vi "pf_Get DLL Path.vi"(8 "error in (no error)":errorcluster) -> (0 "error out":errorcluster, 3 "DLL path":path)   [LabVIEW 2025, in "Photonfocus_Toolkit.lvlib"]
uses:
  Photonfocus_Toolkit.lvlib
  Controls/pf_Toolkit_Error_Type.ctl
  kernel32.dll
panel:
  in  "IWshRuntimeLibrary.IWshShell2":refnum<k7>
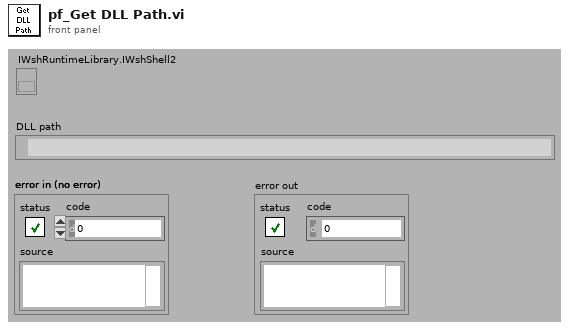
[diagram p1: front panel]
types:
  T1 = typedef "Photonfocus_Toolkit.lvlib/pf_Toolkit_Error_Type.ctl" = enum16{"PF Toolkit_Generic Error", "PF Toolkit_PFConfig Error"}
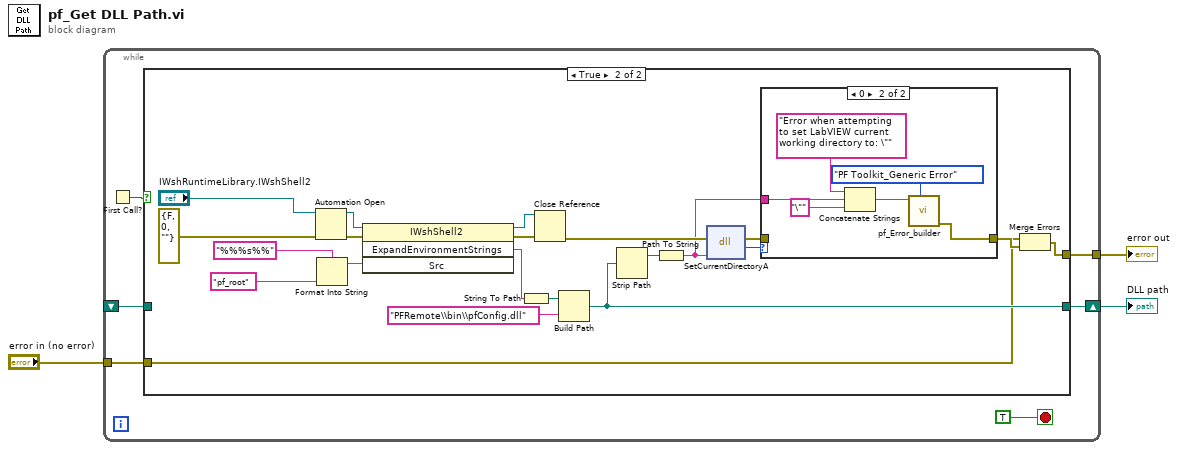
[diagram p0: block diagram]
diagram:
  n1 = while {
    tunnel: "error in (no error)" -> [w8]
    tunnel: [w7] -> w1
    shift-right: [w9] -> w3
    shift-left: _ -> [w5]
    stop <- TRUE stop-if-true
    n2 = First Call?() -> (First Call?: T/F=w4:bool)
    n3 = case shown="True" w4 {
      tunnel: [w11 w20] -> w9
      tunnel: w8 -> [w10 w18]
      tunnel: [w10 w17] -> w7
      tunnel: w5 -> [w11 _]
      frame False {
      }
      frame True {
        n4 = Automation Open(error in (no error)=errorcluster {"status"=FALSE, "code"=0, "source"=""}, Automation Refnum="IWshRuntimeLibrary.IWshShell2") -> (Automation Refnum=w28:refnum<k7>, error out=w31:errorcluster)  [unwired: 2 out]
        n5 = Format Into String(format string="%%%s%%", "pf_root" ("input 1")) -> (resulting string=w26:string)  [unwired: 2 in, 1 out]
        n6 = invoke class="IWshShell2" method="ExpandEnvironmentStrings"(reference=w28, error in=w31, "Src"=w26) -> (reference out=w25:refnum<k7>, error out=w29:errorcluster, "ExpandEnvironmentStrings"=w21:string)  [unwired: 1 in, 1 out]
        n7 = String To Path(string=w21) -> (path=w24:path)
        n8 = Close Reference(reference=w25, error in (no error)=w29) -> (error out=w22:errorcluster)
        n9 = Build Path(base path=w24, name or relative path="PFRemote\\bin\\pfConfig.dll") -> (appended path=w20:path)
        n10 = Strip Path(path=w20) -> (stripped path=w15:path)  [unwired: 1 out]
        n11 = Path To String(path=w15) -> (string=w12:string)
        n12 = dll-call lib="kernel32.dll" fn="SetCurrentDirectoryA"(error in=w22, w12) -> (error out=w13:errorcluster, "return type"=w14:i16)  [unwired: 2 in, 2 out]
        n13 = case shown="0" w14 {
          tunnel: w13 -> [w33 _]
          tunnel: [w33 w36] -> w19
          tunnel: w12 -> [_ w38]
          frame Default {
          }
          frame 0 {
            n14 = Concatenate Strings("Error when attempting to set LabVIEW current working directory to: \"", w38, "\"") -> (w35:string)
            n15 = call "pf_Error_builder.vi"("pf Error Type"=pf_Toolkit_Error_Type."PF Toolkit_Generic Error", "Error message"=w35) -> ("Error cluster out"=w36:errorcluster)  [unwired: 9 out]
          }
        }
        n16 = Merge Errors(w18, w19) -> (w17:errorcluster)
      }
    }
  }
  "DLL path" <- w3
  "error out" <- w1
